vi "energymeter-calibration-wendy.vi"() -> ()   [LabVIEW 2015]
panel:
  out "appended array":dbl[](array[numeric])
  in  "VISA resource -Energy Meter 2":refnum<visa-resource-name>
  in  "VISA resource -Energy Meter":refnum<visa-resource-name>
  in  "# of shots":i32
  in  "stop for shots loop":bool
  out "Current loop #":dbl format="%.4f"
  out "Current Pulse Energy Value Chart":dbl(graph)
  out "Current Pulse Energy Value":dbl=5.0 caption="Value"
  out "Current Pulse Energy Value Chart 2":dbl(graph)
  out "Current Pulse Energy Value 2":dbl=5.0 caption="Value"
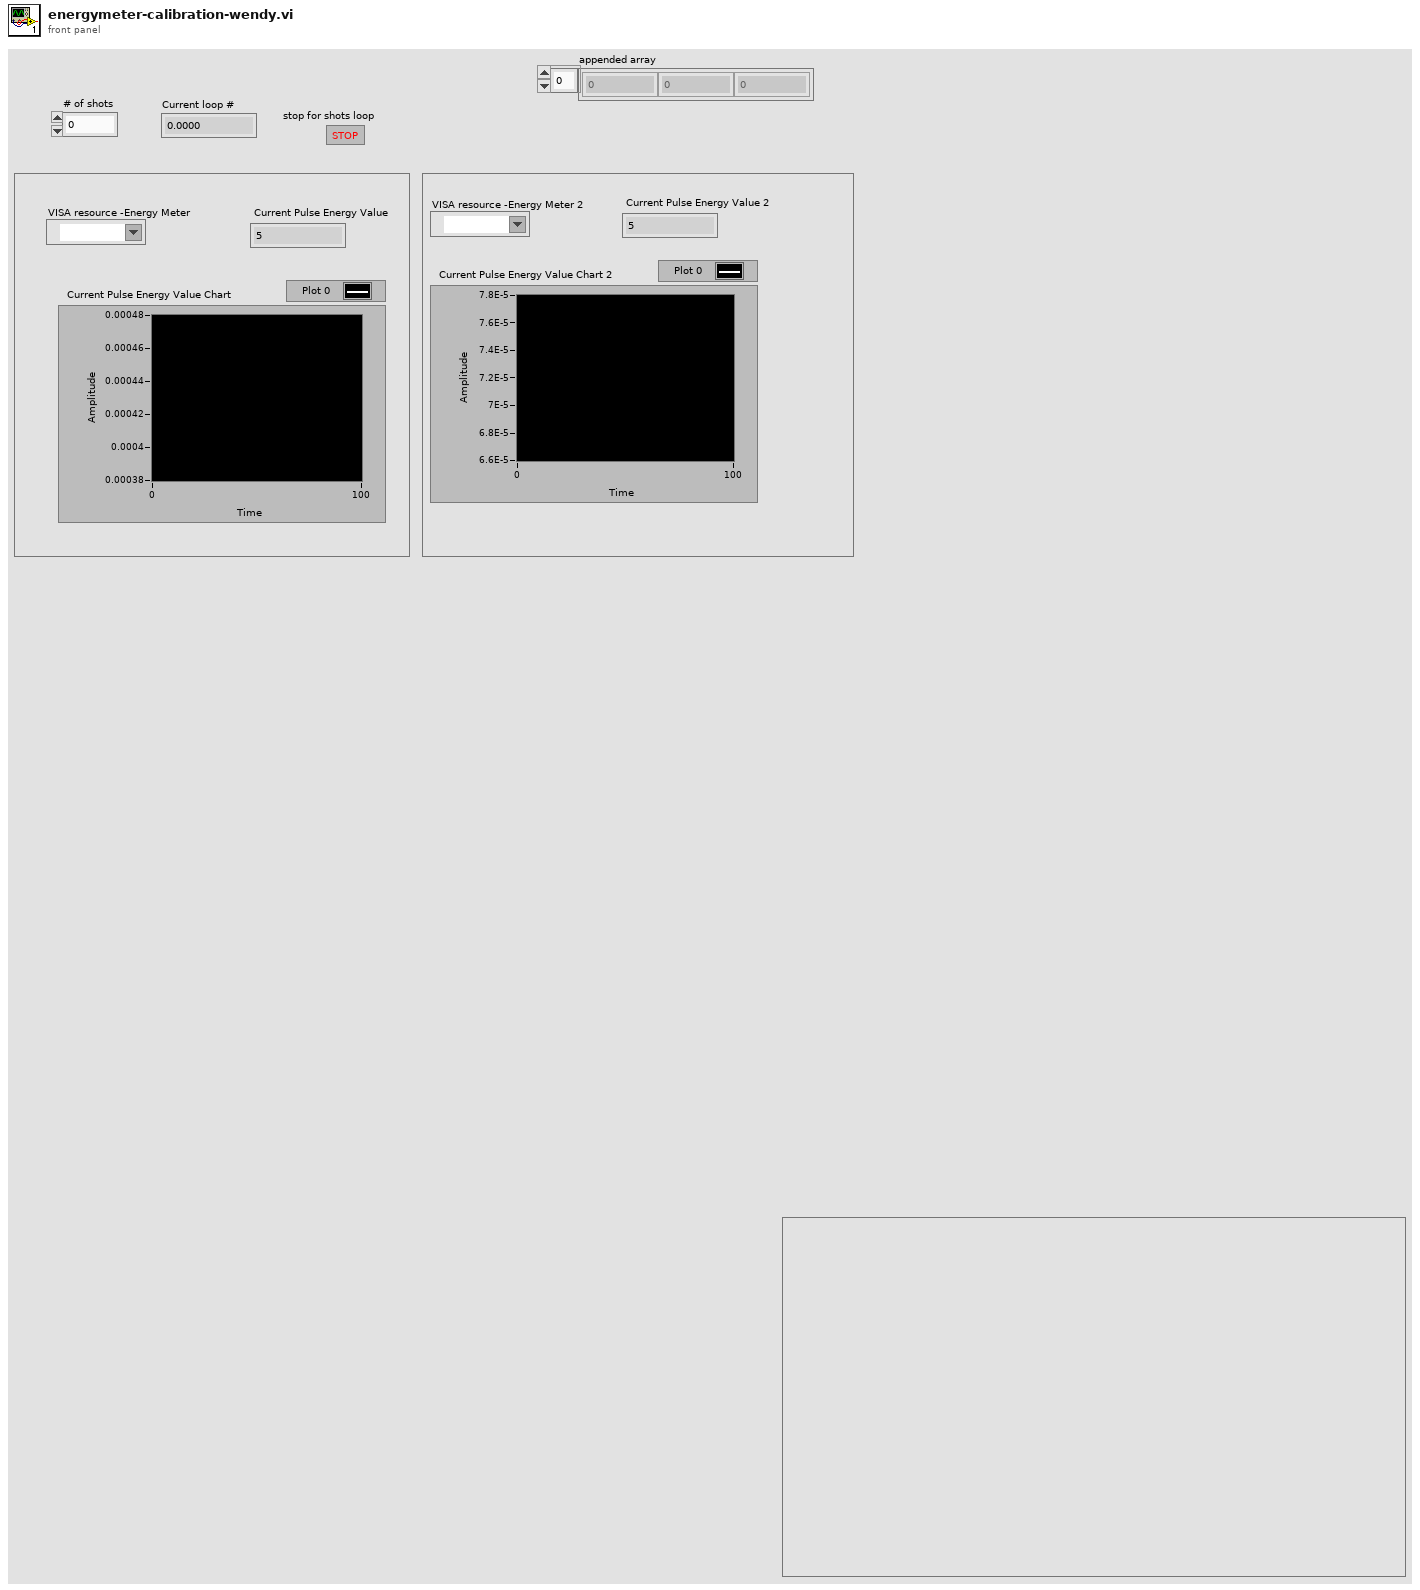
[diagram p1: front panel]
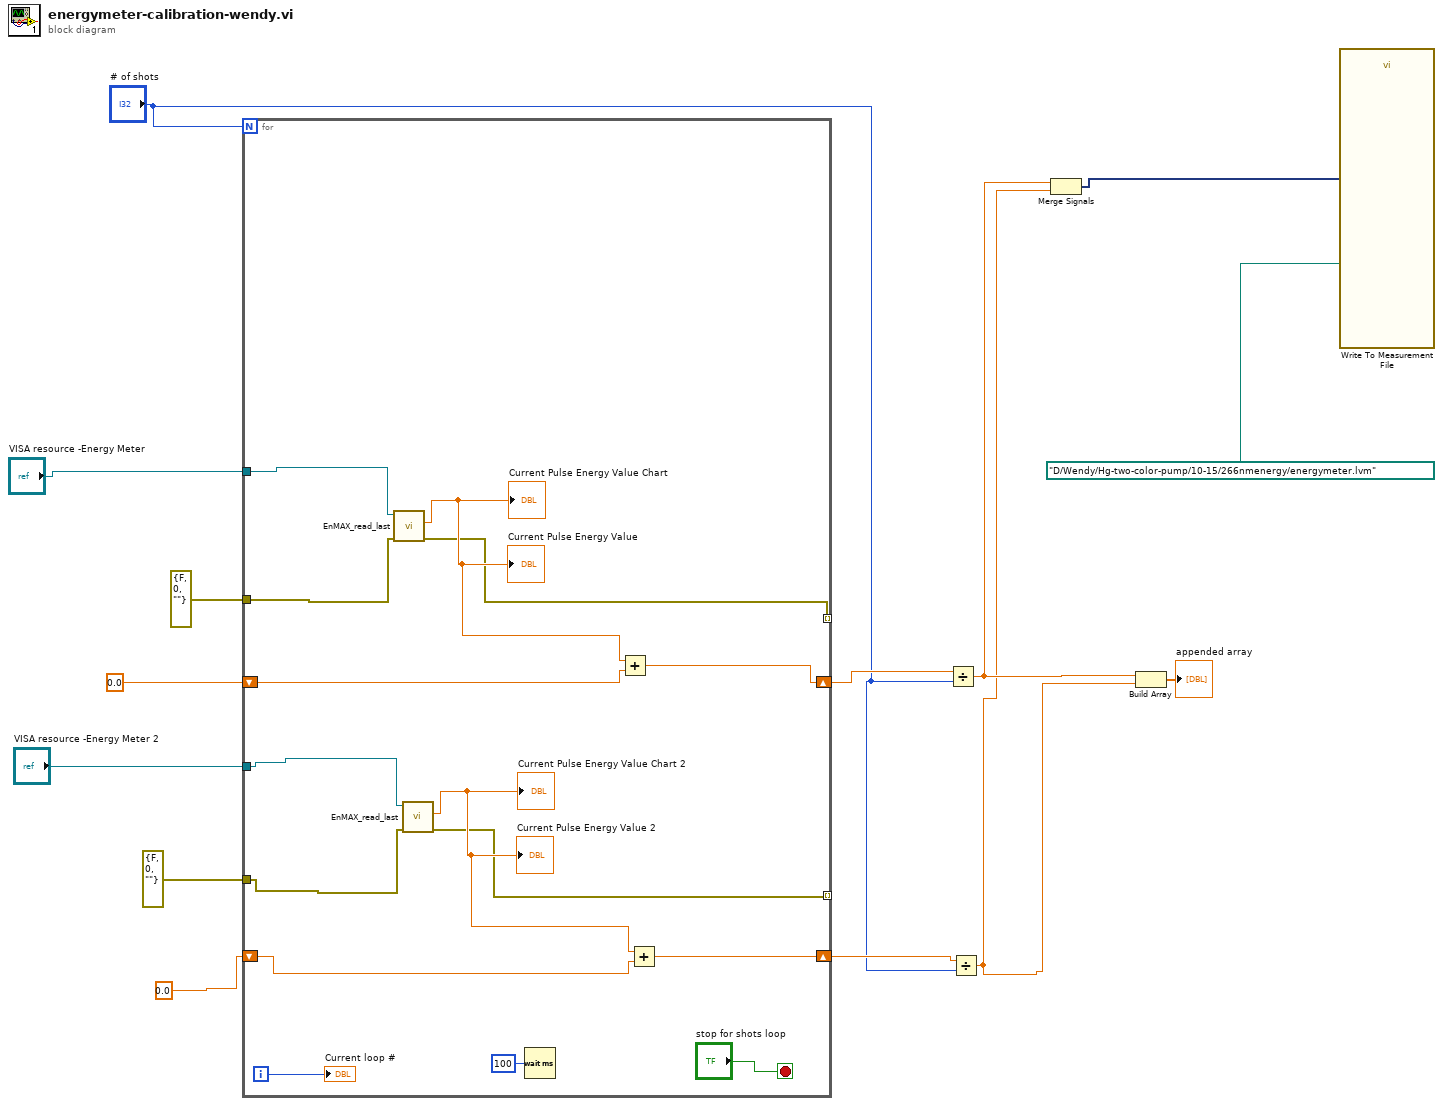
[diagram p0: block diagram]
diagram:
  n1 = for {
    N: "# of shots" -> [_]
    tunnel: "VISA resource -Energy Meter" -> [w26]
    tunnel: errorcluster {"status"=FALSE, "code"=0, "source"=""} ("error in (no error)") -> [w25]
    shift-right: [w22] -> w11
    shift-left: 0.0 ("y") -> [w23]
    tunnel: [w21] -> _ mode=indexing
    tunnel: "VISA resource -Energy Meter 2" -> [w19]
    tunnel: errorcluster {"status"=FALSE, "code"=0, "source"=""} ("error in (no error)") -> [w18]
    tunnel: [w17] -> _ mode=indexing
    shift-right: [w16] -> w5
    shift-left: 0.0 ("y") -> [w15]
    i -> [w28]
    stop <- "stop for shots loop" stop-if-true
    n2 = call "EnMAX_read_last.vi"("error in"=w25, "VISA in"=w26) -> ("error out"=w21:errorcluster, "Value"=w24:dbl)  [unwired: 7 in, 1 out]
    "Current Pulse Energy Value Chart" <- w24
    "Current Pulse Energy Value" <- w24
    n3 = call "EnMAX_read_last.vi"("error in"=w18, "VISA in"=w19) -> ("error out"=w17:errorcluster, "Value"=w20:dbl)  [unwired: 7 in, 1 out]
    "Current Pulse Energy Value Chart 2" <- w20
    "Current Pulse Energy Value 2" <- w20
    n4 = Wait (ms)(milliseconds to wait=u32 100) -> ()  [unwired: 1 out]
    n5 = Add(x=w24, y=w23) -> (x+y=w22:dbl)
    n6 = Add(x=w20, y=w15) -> (x+y=w16:dbl)
    "Current loop #" <- w28
  }
  n7 = Divide(x=w11, y="# of shots") -> (x/y=w3:dbl)
  n8 = Divide(x=w5, y="# of shots") -> (x/y=w2:dbl)
  n9 = Merge Signals(w3, w2) -> (w9:dynamicdata)
  n10 = Build Array(w3, w2) -> (→"appended array":dbl[])
  n11 = call "Write To Measurement File"("Signals"=w9, "Filename"=path "D:/Wendy/Hg-two-color-pump/10-15/266nmenergy/energymeter.lvm") -> ()  [unwired: 15 in, 3 out]
